vi "Test GenNet-Server API.vi"() -> ()   [LabVIEW 2020]
doc: "GenNet-Server API Tester.\n\n____\nHAMPEL SOFTWARE ENGINEERING v3.8.0 (2023-12-18 14:41)"
uses:
  UDP Broadcasting/Network Broadcast Params.ctl
  <vilib>/Utility/error.llb/DialogType.ctl
  DQMH-GenNet Message Queue.lvclass
  UDP Broadcasting/Generic Broadcasts.ctl
  hse-dqmh/Dynamic Requesters/Singleton/Status Updated Argument--cluster.ctl
  hse-dqmh/Dynamic Requesters/Singleton/Error Reported Argument--cluster.ctl
  hse-dqmh/Dynamic Requesters/Singleton/Get Module Execution Status Argument--cluster.ctl
  hse-dqmh/Dynamic Requesters/Singleton/Stop Argument--cluster.ctl
  hse-dqmh/Controls/System Message Argument--cluster.ctl
  hse-dqmh/Controls/System Message Source.ctl
  GenNet-Server.lvlib
  hse-dqmh/hse-dqmh-dynamicrequesters.lvlib
  hse-dqmh/hse-dqmh.lvlib
  hse-gennet.lvlib
panel:
  out "last error":errorcluster
  in  "Show Main VI Diagram on Init (F)":bool
  in  "UDP Connection Parameters":T1
  in  "Forward Generic Broadcasts to Network":bool
  in  "Port Number":u16
  in  "Run as Singleton?":bool
  in  "Show Block Diagram":bool
  in  "Refresh Modules":bool
  out "Active Modules":string[](array[string])
  in  "Stop Module":bool
  in  "Select Module":i32(ring)=-1 caption="Select Module\nTo send Request to" items=["All"=-1]
  in  "Run New Module":bool
  in  "Hide Module Panel":bool
  in  "Show Module Panel":bool
  out "Status":string
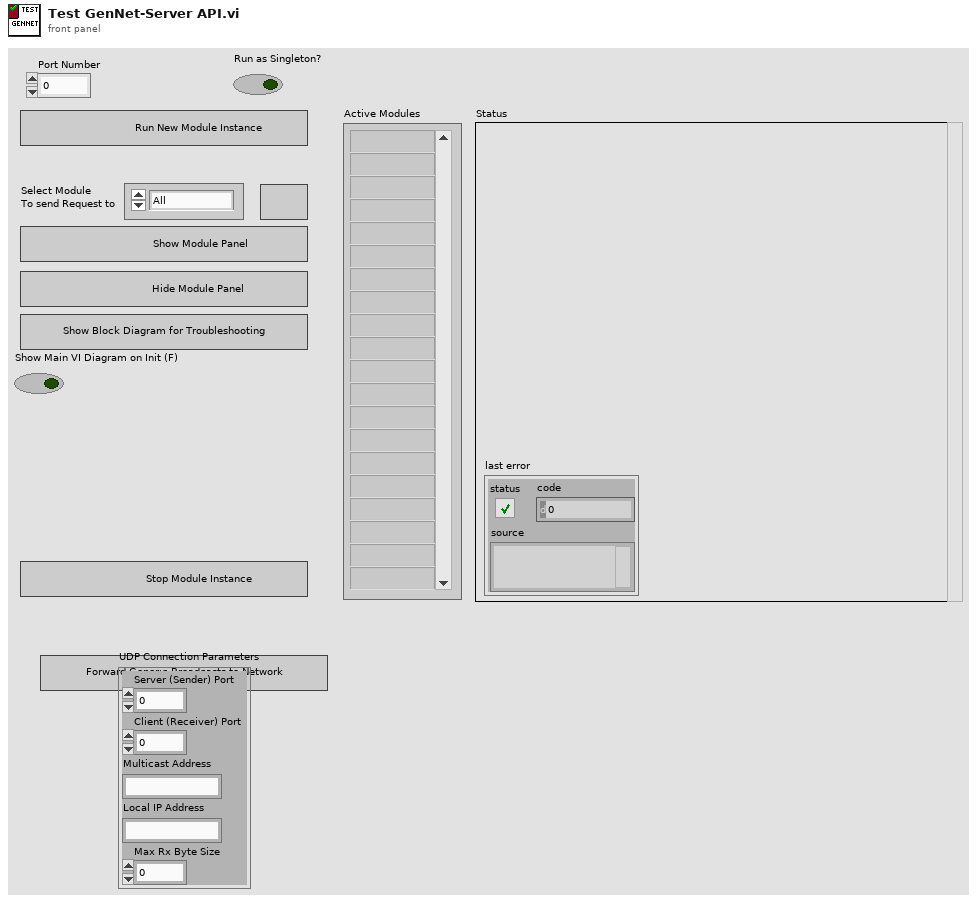
[diagram p1: front panel]
types:
  T1 = typedef "hse-gennet.lvlib/Network Broadcast Params.ctl" = cluster{"Server (Sender) Port":u16, "Client (Receiver) Port":u16, "Multicast Address":string, "Local IP Address":string, "Max Rx Byte Size":i32}
  T2 = typedef "GenNet-Server.lvlib/Broadcast Events--cluster.ctl" = cluster{"Module Did Init":refnum<user-event>, "Status Updated":refnum<user-event>, "Error Reported":refnum<user-event>, "Module Did Stop":refnum<user-event>, "Update Module Execution Status":refnum<user-event>, "GenNet Message Received":refnum<user-event>}
  T3 = typedef "DialogType.ctl" = u16
  T4 = typedef "hse-gennet.lvlib/Generic Broadcasts.ctl" = cluster{"Status Updated":refnum<user-event>, "Error Reported":refnum<user-event>, "Update Module Execution Status":refnum<user-event>, "Module Did Stop":refnum<user-event>, "System Message":refnum<user-event>}
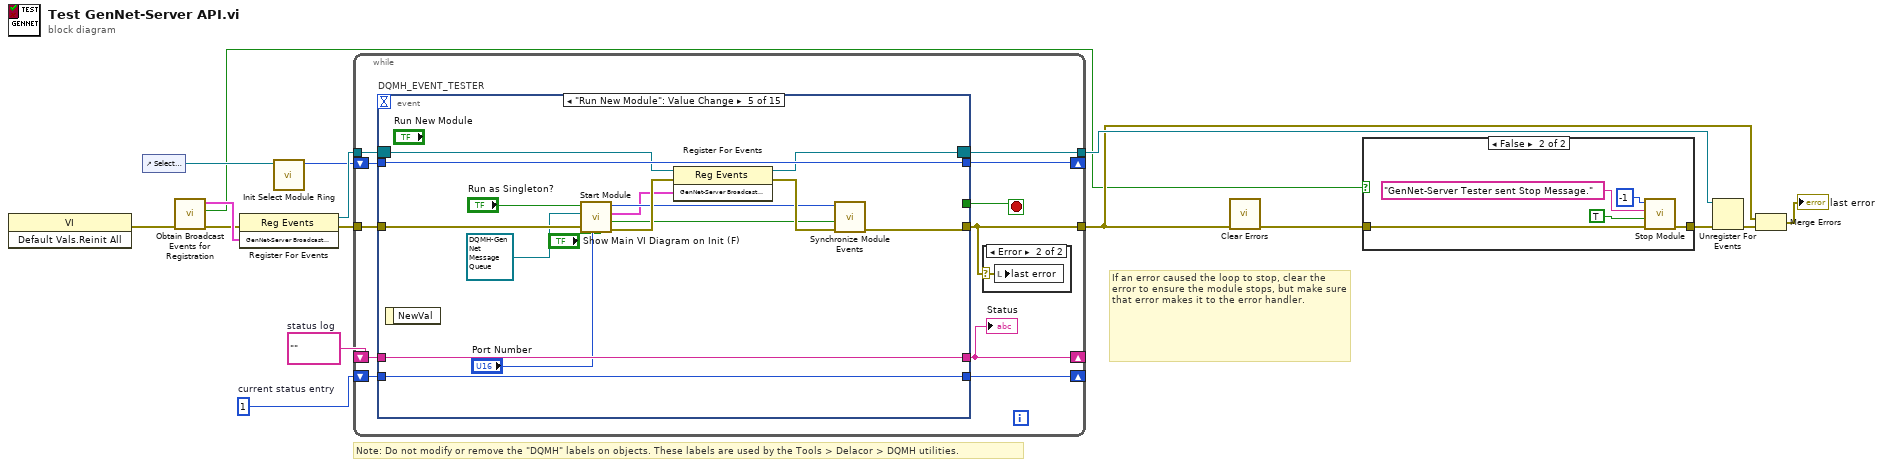
[diagram p0: block diagram]
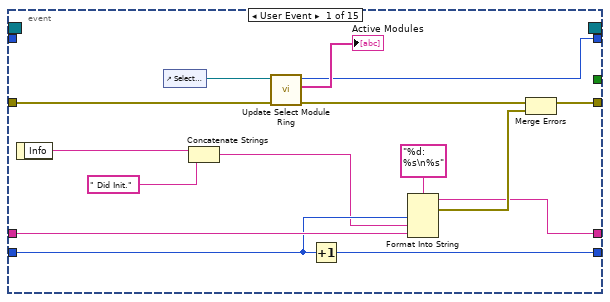
[diagram p4: hidden frame]
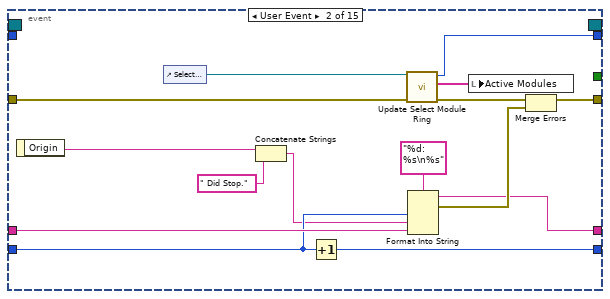
[diagram p5: hidden frame]
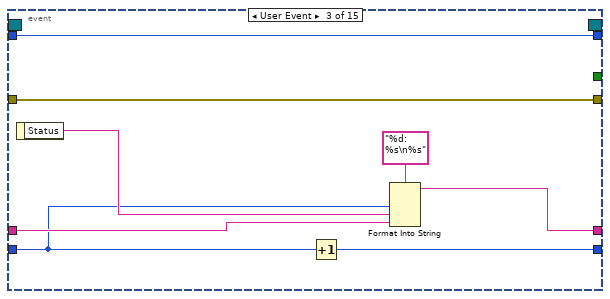
[diagram p6: hidden frame]
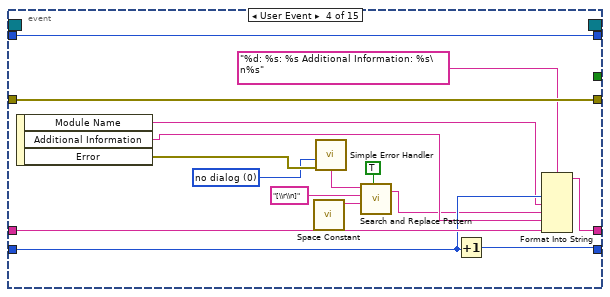
[diagram p7: hidden frame]
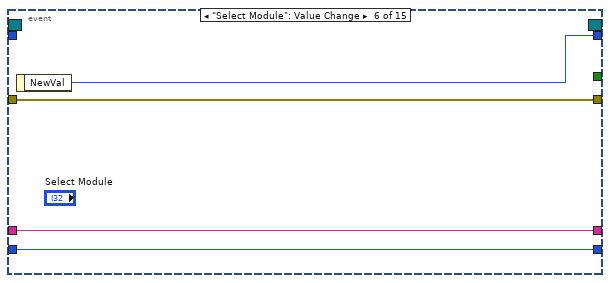
[diagram p8: hidden frame]
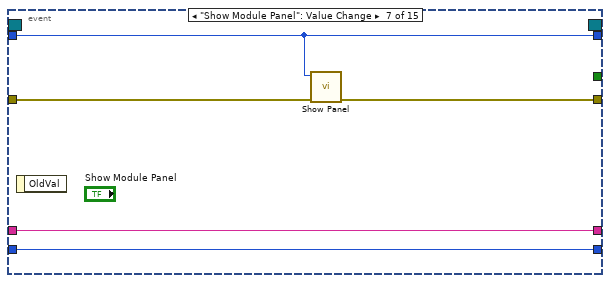
[diagram p9: hidden frame]
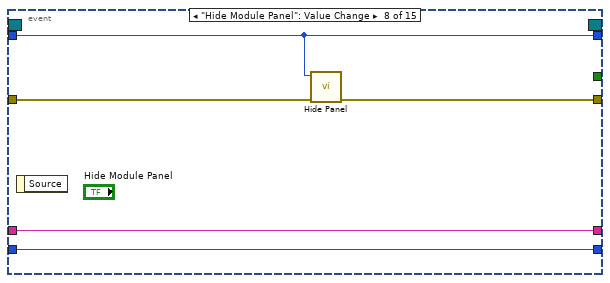
[diagram p10: hidden frame]
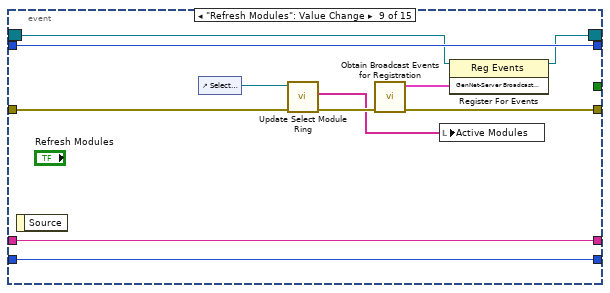
[diagram p11: hidden frame]
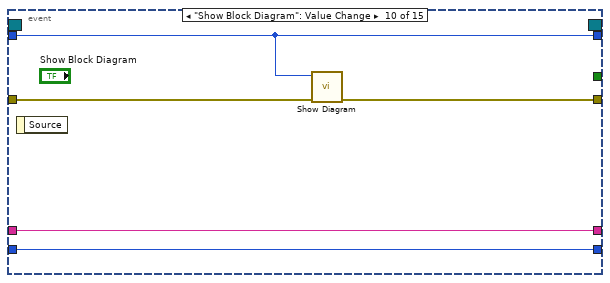
[diagram p12: hidden frame]
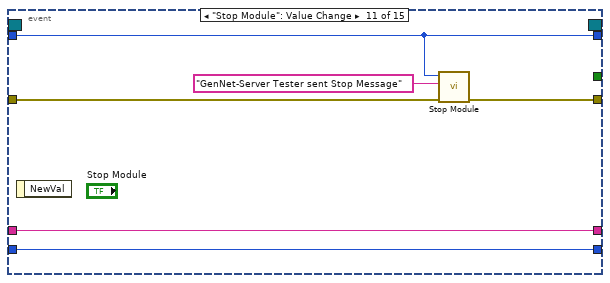
[diagram p13: hidden frame]
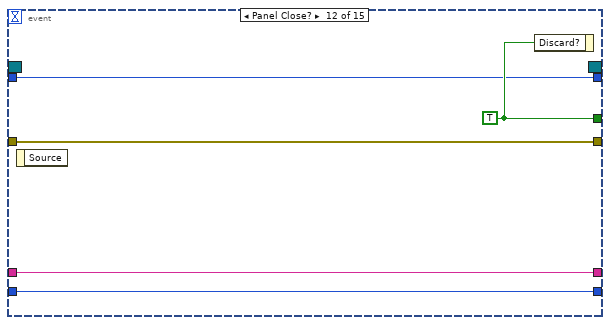
[diagram p14: hidden frame]
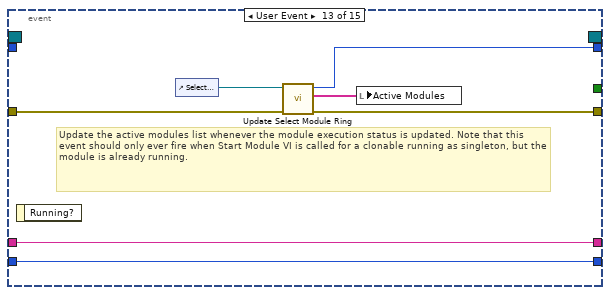
[diagram p15: hidden frame]
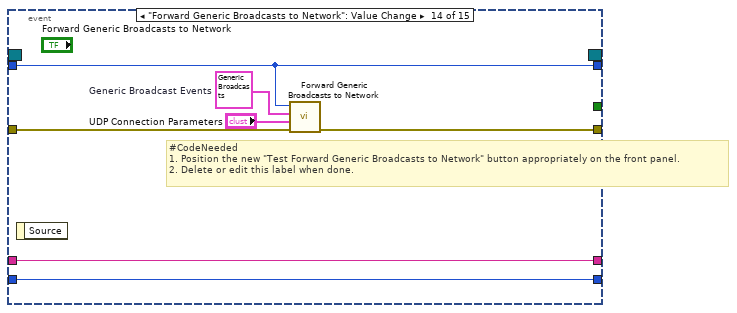
[diagram p16: hidden frame]
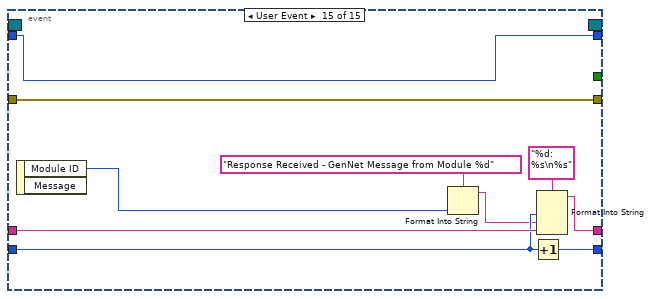
[diagram p17: hidden frame]
diagram:
  w12 = 1  # current status entry
  w13 = ""  # status log
  # "If an error caused the loop to stop, clear the error to ensure the module stops, but make sure that error makes it to the error handler."
  # "Note: Do not modify or remove the \"DQMH\" labels on objects. These labels are used by the Tools > Delacor > DQMH utilities."
  n1 = invoke class="VI" method="Default Vals.Reinit All"() -> (error out=w4:errorcluster)  [unwired: 3 in, 2 out]
  n2 = control-ref of="Select Module"() -> (w10:refnum<vi>)
  n3 = call "Obtain Broadcast Events for Registration.vi"("error in (no error)"=w4) -> ("error out"=w3:errorcluster, "Already running?"=w2:bool, "GenNet-Server Broadcast Events"=w9:T2)  [unwired: 8 in]
  n4 = register-events(error in=w3, w9) -> (reference out=w16:refnum<event-registration>, error out=w8:errorcluster)  [unwired: 1 in]
  n5 = call "Init Select Module Ring.vi"("Select Module Ring Ref"=w10) -> ("Value for All Modules"=w11:i32)  [unwired: 8 in, 2 out]
  n6 = while {
    tunnel: w16 -> [w27]
    tunnel: [w18] -> w5
    tunnel: w8 -> [w26]
    shift-right: [w22] -> _
    shift-left: w13 -> [w24]
    shift-right: [w23] -> _
    shift-left: w12 -> [w25]
    shift-right: [w20] -> _
    shift-left: w11 -> [w21]
    tunnel: [w19] -> w7
    stop <- w17 stop-if-true
    n7 = event "DQMH_EVENT_TESTER" shown="[4] \"Run New Module\": Value Change" {
      selector: w27 -> [_ _ _ _ w92 _ _ _ w118 _ _ _ _ _ _]
      dyn-events: [_ _ _ _ w91 _ _ _ w117 _ _ _ _ _ _] -> w19
      timeout: _ -> [_ _ _ _ _ _ _ _ _ _ _ _ _ _ _]
      tunnel: [_ _ _ _ _ _ _ _ _ _ _ w139 _ _ _] -> w17
      tunnel: [w32 w50 w66 w81 w90 w102 w106 w111 w114 w125 w130 w138 w142 w150 w163] -> w18
      tunnel: w26 -> [w34 w52 w66 w81 w93 w102 w107 w112 w119 w128 w131 w138 w143 w153 w163]
      tunnel: w25 -> [w40 w55 w59 w78 w95 w100 w104 w109 w122 w126 w133 w136 w145 w151 w159]
      tunnel: w24 -> [w41 w56 w62 w80 w96 w101 w105 w110 w123 w127 w134 w137 w146 w152 w161]
      tunnel: [w38 w53 w63 w79 w96 w101 w105 w110 w123 w127 w134 w137 w146 w152 w160] -> w22
      tunnel: [w39 w54 w65 w77 w95 w100 w104 w109 w122 w126 w133 w136 w145 w151 w158] -> w23
      tunnel: w21 -> [_ _ w60 w82 w94 _ w103 w108 w121 w124 w132 w135 _ w149 w162]
      tunnel: [w29 w47 w60 w82 w94 w99 w103 w108 w121 w124 w132 w135 w141 w149 w162] -> w20
      event User Event {
        n8 = event-data() -> ("Info"=w37:string)  [unwired: 1 in]
        n9 = control-ref of="Select Module"() -> (w31:refnum<vi>)
        n10 = Concatenate Strings(w37, " Did Init.") -> (w36:string)
        n11 = call "Update Select Module Ring.vi"("error in (no error)"=w34, "Select Module Ring Ref"=w31) -> ("error out"=w33:errorcluster, "Active Modules (Array)"=→"Active Modules":string[], "New Module Ring Value"=w29:i32)  [unwired: 7 in]
        n12 = Increment(x=w40) -> (x+1=w39:i32)
        n13 = Format Into String(format string="%d: %s\n%s", w40, w36, w41) -> (resulting string=w38:string, error out=w43:errorcluster)  [unwired: 2 in]
        n14 = Merge Errors(w33, w43) -> (w32:errorcluster)
      }
      event User Event {
        n15 = event-data() -> ("Origin"=w45:string)  [unwired: 1 in]
        n16 = control-ref of="Select Module"() -> (w49:refnum<vi>)
        n17 = Concatenate Strings(w45, " Did Stop.") -> (w44:string)
        n18 = Increment(x=w55) -> (x+1=w54:i32)
        n19 = call "Update Select Module Ring.vi"("error in (no error)"=w52, "Select Module Ring Ref"=w49) -> ("error out"=w51:errorcluster, "Active Modules (Array)"=w48:string[], "New Module Ring Value"=w47:i32)  [unwired: 7 in]
        n20 = Format Into String(format string="%d: %s\n%s", w55, w44, w56) -> (resulting string=w53:string, error out=w58:errorcluster)  [unwired: 2 in]
        n21 = local write "Active Modules"(w48) -> ()
        n22 = Merge Errors(w51, w58) -> (w50:errorcluster)
      }
      event User Event {
        n23 = event-data() -> ("Status"=w61:string)  [unwired: 1 in]
        n24 = Increment(x=w59) -> (x+1=w65:i32)
        n25 = Format Into String(format string="%d: %s\n%s", w59, w61, w62) -> (resulting string=w63:string)  [unwired: 2 in, 1 out]
      }
      event User Event {
        w73 = T3 0 items=["no dialog", "OK message", "continue or stop message", "OK message + warnings", "continue/stop + warnings"] ("type of dialog (OK msg:1)")
        n26 = event-data() -> ("Module Name"=w74:string, "Additional Information"=w75:string, "Error"=w76:errorcluster)  [unwired: 1 in]
        n27 = call <vilib>:"Space Constant.vi"() -> ("String"=w69:string)
        n28 = call <vilib>:"Simple Error Handler.vi"("type of dialog (OK msg:1)"=w73, "error in (no error)"=w76) -> ("message"=w72:string)  [unwired: 3 in, 4 out]
        n29 = call <vilib>:"Search and Replace Pattern.vi"("string"=w72, "regular expression (\"\")"="[\\r\\n]" ("regular expression (\"\")"), "replace string (\"\")"=w69, "replace all? (F)"=TRUE ("replace all CR/LF with spaces")) -> ("result string"=w71:string)  [unwired: 1 in, 1 out]
        n30 = Increment(x=w78) -> (x+1=w77:i32)
        n31 = Format Into String(format string="%d: %s: %s Additional Information: %s\n%s", w78, w74, w71, w75, w80) -> (resulting string=w79:string)  [unwired: 2 in, 1 out]
      }
      event "Run New Module": Value Change {
        n32 = event-data() -> ()  [unwired: 1 in, 1 out]
        n33 = call "Start Module.vi"("Show Main VI Diagram on Init (F)"="Show Main VI Diagram on Init (F)", "Port Number"="Port Number", "error in (no error)"=w93, "Caller MsgQ"=refnum<class "DQMH-GenNet Message Queue.lvclass"> refnum, "Run as Singleton? (F)"="Run as Singleton?") -> ("error out"=w97:errorcluster, "Wait for Event Sync?"=w88:bool, "GenNet-Server Broadcast Events"=w87:T2, "Module ID"=w89:i32)  [unwired: 3 in]
        n34 = register-events(reference=w92, error in=w97, w87) -> (reference out=w91:refnum<event-registration>, error out=w98:errorcluster)
        n35 = call "Synchronize Module Events.vi"("error in (no error)"=w98, "Wait for Event Sync?"=w88, "Module ID"=w89) -> ("error out"=w90:errorcluster)  [unwired: 7 in, 1 out]
      }
      event "Select Module": Value Change {
        n36 = event-data() -> ("NewVal"=w99:i32)  [unwired: 1 in]
      }
      event "Show Module Panel": Value Change {
        n37 = event-data() -> ()  [unwired: 1 in, 1 out]
        n38 = call "Show Panel.vi"("error in (no error)"=w107, "Module ID"=w103) -> ("error out"=w106:errorcluster)  [unwired: 9 in]
      }
      event "Hide Module Panel": Value Change {
        n39 = event-data() -> ()  [unwired: 1 in, 1 out]
        n40 = call "Hide Panel.vi"("error in (no error)"=w112, "Module ID"=w108) -> ("error out"=w111:errorcluster)  [unwired: 9 in]
      }
      event "Refresh Modules": Value Change {
        n41 = event-data() -> ()  [unwired: 1 in, 1 out]
        n42 = control-ref of="Select Module"() -> (w120:refnum<vi>)
        n43 = call "Update Select Module Ring.vi"("error in (no error)"=w119, "Select Module Ring Ref"=w120) -> ("error out"=w115:errorcluster, "Active Modules (Array)"=w113:string[])  [unwired: 7 in, 1 out]
        n44 = call "Obtain Broadcast Events for Registration.vi"("error in (no error)"=w115) -> ("error out"=w114:errorcluster, "GenNet-Server Broadcast Events"=w116:T2)  [unwired: 8 in, 1 out]
        n45 = local write "Active Modules"(w113) -> ()
        n46 = register-events(reference=w118, w116) -> (reference out=w117:refnum<event-registration>)  [unwired: 1 in, 1 out]
      }
      event "Show Block Diagram": Value Change {
        n47 = event-data() -> ()  [unwired: 1 in, 1 out]
        n48 = call "Show Diagram.vi"("error in (no error)"=w128, "Module ID"=w124) -> ("error out"=w125:errorcluster)  [unwired: 9 in]
      }
      event "Stop Module": Value Change {
        n49 = event-data() -> ()  [unwired: 1 in, 1 out]
        n50 = call "Stop Module.vi"("error in (no error)"=w131, "Origin"="GenNet-Server Tester sent Stop Message", "Module ID"=w132) -> ("error out"=w130:errorcluster)  [unwired: 8 in]
      }
      event Panel Close? {
        w139 = TRUE ("Discard?")
        n51 = event-data() -> ()  [unwired: 1 in, 1 out]
        n52 = event-data("Discard?"=w139) -> ()  [unwired: 1 in, 1 out]
      }
      event User Event {
        # "Update the active modules list whenever the module execution status is updated. Note that this event should only ever fire when Start Module VI is called for a clonable running as singleton, but the module is already running."
        n53 = event-data() -> ()  [unwired: 1 in, 1 out]
        n54 = control-ref of="Select Module"() -> (w144:refnum<vi>)
        n55 = call "Update Select Module Ring.vi"("error in (no error)"=w143, "Select Module Ring Ref"=w144) -> ("error out"=w142:errorcluster, "Active Modules (Array)"=w140:string[], "New Module Ring Value"=w141:i32)  [unwired: 7 in]
        n56 = local write "Active Modules"(w140) -> ()
      }
      event "Forward Generic Broadcasts to Network": Value Change {
        w147 = T4 {"Status Updated"=refnum, "Error Reported"=refnum, "Update Module Execution Status"=refnum, "Module Did Stop"=refnum, "System Message"=refnum}  # Generic Broadcast Events
        # "#CodeNeeded\n1. Position the new \"Test Forward Generic Broadcasts to Network\" button appropriately on the front panel.\n2. Delete or edit this label when done."
        n57 = event-data() -> ()  [unwired: 1 in, 1 out]
        n58 = call "Forward Generic Broadcasts to Network.vi"("error in (no error)"=w153, "Network Broadcast Params"="UDP Connection Parameters", "Generic Broadcast Events"=w147, "Module ID"=w149) -> ("error out"=w150:errorcluster)  [unwired: 7 in]
      }
      event User Event {
        n59 = event-data() -> ("Module ID"=w154:i32)  [unwired: 1 in, 1 out]
        n60 = Format Into String(format string="Response Received - GenNet Message from Module %d", w154) -> (resulting string=w155:string)  [unwired: 2 in, 1 out]
        n61 = Increment(x=w159) -> (x+1=w158:i32)
        n62 = Format Into String(format string="%d: %s\n%s", w159, w155, w161) -> (resulting string=w160:string)  [unwired: 2 in, 1 out]
      }
    }
    "Status" <- w22
    n63 = case "DQMH_TESTER_ERROR_LOCAL" shown="Error" w18 {
      selector: w18 -> [_ w28]
      frame No Error {
      }
      frame Error {
        n64 = local write "last error"(w28) -> ()
      }
    }
  }
  n65 = call <vilib>:"Clear Errors.vi"("error in (no error)"=w5) -> ("error out"=w6:errorcluster)  [unwired: 5 in, 1 out]
  n66 = case shown="False" w2 {
    tunnel: [w164 w169] -> w14
    tunnel: w6 -> [w164 w166]
    frame True {
    }
    frame False {
      n67 = call "Stop Module.vi"("error in (no error)"=w166, "Wait for Module to stop? (F)"=TRUE ("Wait for Module to stop?"), "Origin"="GenNet-Server Tester sent Stop Message.", "Module ID"=-1) -> ("error out"=w169:errorcluster)  [unwired: 7 in]
    }
  }
  n68 = Unregister For Events(event registration refnum=w7, error in=w14) -> (error out=w15:errorcluster)
  n69 = Merge Errors(w5, w15) -> (→"last error":errorcluster)
